vi "MSScript_SubVI_IsARegularVariable.vi"(9 "VarString in":string) -> (1 "Variable simbol no found":bool, 2 "irregular":bool, 3 "VarString out":string)   [LabVIEW 2018, in "MSScript.lvclass"]
uses:
  MSScript.lvclass
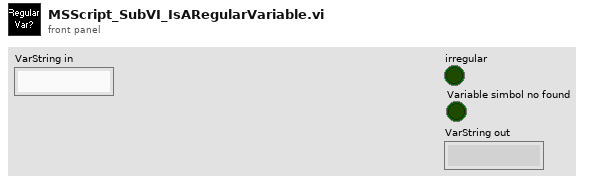
[diagram p1: front panel]
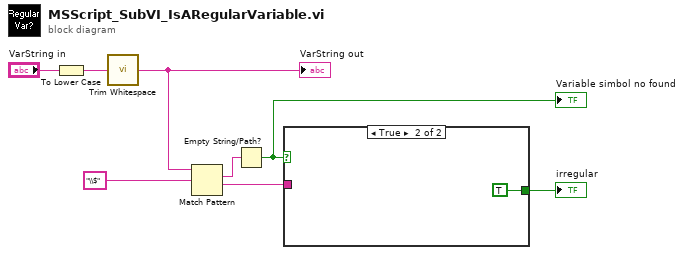
[diagram p0: block diagram]
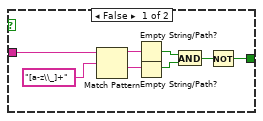
[diagram p2: hidden frame]
diagram:
  n1 = To Lower Case(string="VarString in") -> (all lower case string=w2:string)
  n2 = call <vilib>:"Trim Whitespace.vi"("string"=w2) -> ("trimmed string"=w1:string)  [unwired: 1 in]
  "VarString out" <- w1
  n3 = Match Pattern(string=w1, regular expression="\\$") -> (match substring=w7:string, after substring=w6:string)  [unwired: 1 in, 2 out]
  n4 = Empty String/Path?(string/path=w7) -> (empty?=w3:bool)
  "Variable simbol no found" <- w3
  n5 = case shown="True" w3 {
    tunnel: [w10 TRUE] -> w4
    tunnel: w6 -> [w9 _]
    frame False {
      n6 = Match Pattern(string=w9, regular expression="[a-z\\_]+") -> (before substring=w15:string, after substring=w14:string)  [unwired: 1 in, 2 out]
      n7 = Empty String/Path?(string/path=w15) -> (empty?=w13:bool)
      n8 = Empty String/Path?(string/path=w14) -> (empty?=w12:bool)
      n9 = And(x=w13, y=w12) -> (x .and. y?=w11:bool)
      n10 = Not(x=w11) -> (.not. x?=w10:bool)
    }
    frame True {
    }
  }
  "irregular" <- w4
